vi "Read Motor Velocity.vi"(8 "error in (no error)":errorcluster, 10 "Motor ID (0)":u8, 11 "VISA resource name":refnum<visa-resource-name>) -> (0 "error out":errorcluster, 2 "Velocity (RPM)":dbl, 3 "VISA resource name out":refnum<visa-resource-name>)   [LabVIEW 2016, in "Dynamixel Motor.lvlib"]
doc: "Retrieves the motor's velocity."
uses:
  Dynamixel Motor.lvlib
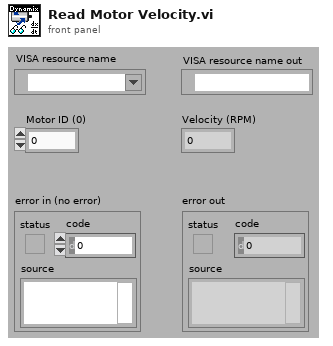
[diagram p1: front panel]
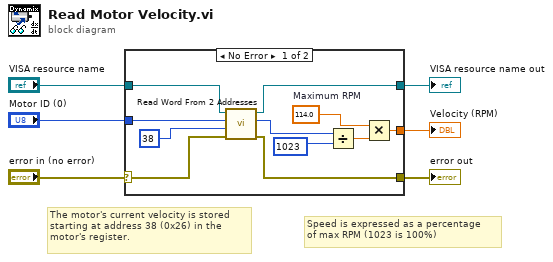
[diagram p0: block diagram]
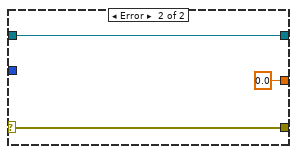
[diagram p2: hidden frame]
diagram:
  # "The motor's current velocity is stored\nstarting at address 38 (0x26) in the\nmotor's register."
  # "Speed is expressed as a percentage \nof max RPM (1023 is 100%)"
  n1 = case shown="No Error" "error in (no error)" {
    selector: "error in (no error)" -> [w7 w19]
    tunnel: "VISA resource name" -> [w16 w20]
    tunnel: [w15 w20] -> w5
    tunnel: [w14 w19] -> w4
    tunnel: [w11 0.0] -> w3
    tunnel: "Motor ID (0)" -> [w9 _]
    frame No Error {
      w10 = 114.0  # Maximum RPM
      n2 = call "Read Word From 2 Addresses.vi"("Error in (no error)"=w7, "Address number (0)"=u8 38 ("Address # DEC"), "Motor ID (0)"=w9, "VISA resource name"=w16) -> ("error out"=w14:errorcluster, "Data"=w17:u16, "VISA resource name out"=w15:refnum<visa-resource-name>)  [unwired: 5 in]
      n3 = Divide(x=w17, y=1023) -> (x/y=w12:dbl)
      n4 = Multiply(x=w10, y=w12) -> (x*y=w11:dbl)
    }
    frame Error {
    }
  }
  "VISA resource name out" <- w5
  "error out" <- w4
  "Velocity (RPM)" <- w3
